vi "loadEthernetRange.vi"(6 "type":string, 8 "error in (no error)":errorcluster, 9 "device.lvclass":refnum<class "device.lvclass">, 10 "xml in":refnum<class "NativeXML.lvclass">, 11 "deviceDataBase in":refnum<class "deviceDataBase.lvclass">) -> (0 "error out":errorcluster, 1 "device.lvclass out":refnum<class "device.lvclass">, 2 "xml out":refnum<class "NativeXML.lvclass">, 3 "deviceDataBase out":refnum<class "deviceDataBase.lvclass">)   [LabVIEW 2011, in "Tools.lvlib" / "DatabaseHelpers.lvlib" / "deviceDataBase.lvclass"]
uses:
  deviceDataBase.lvclass
  NativeXML/NativeXML.lvclass
  Database Objects/device/device.lvclass
  Database Objects/device/EthernetSupply/ethernetSupply.lvclass
  Database Objects/device/AnalogDevice/AnalogDevice.lvclass
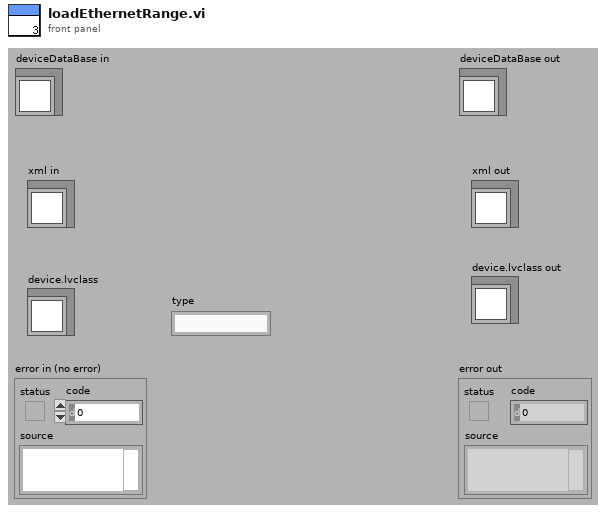
[diagram p1: front panel]
types:
  T1 = cluster{"Range":cluster{"units":string, "current":dbl, "voltage":dbl}, "triggering_inUse":cluster{"start_trigger":string, "clock":string}, "Limits":cluster{"VoltageLimit":dbl, "CurrentLimit":dbl}}[]
  T2 = cluster{"Range":cluster{"units":string, "current":dbl, "voltage":dbl}, "triggering_inUse":cluster{"start_trigger":string, "clock":string}, "Limits":cluster{"VoltageLimit":dbl, "CurrentLimit":dbl}}
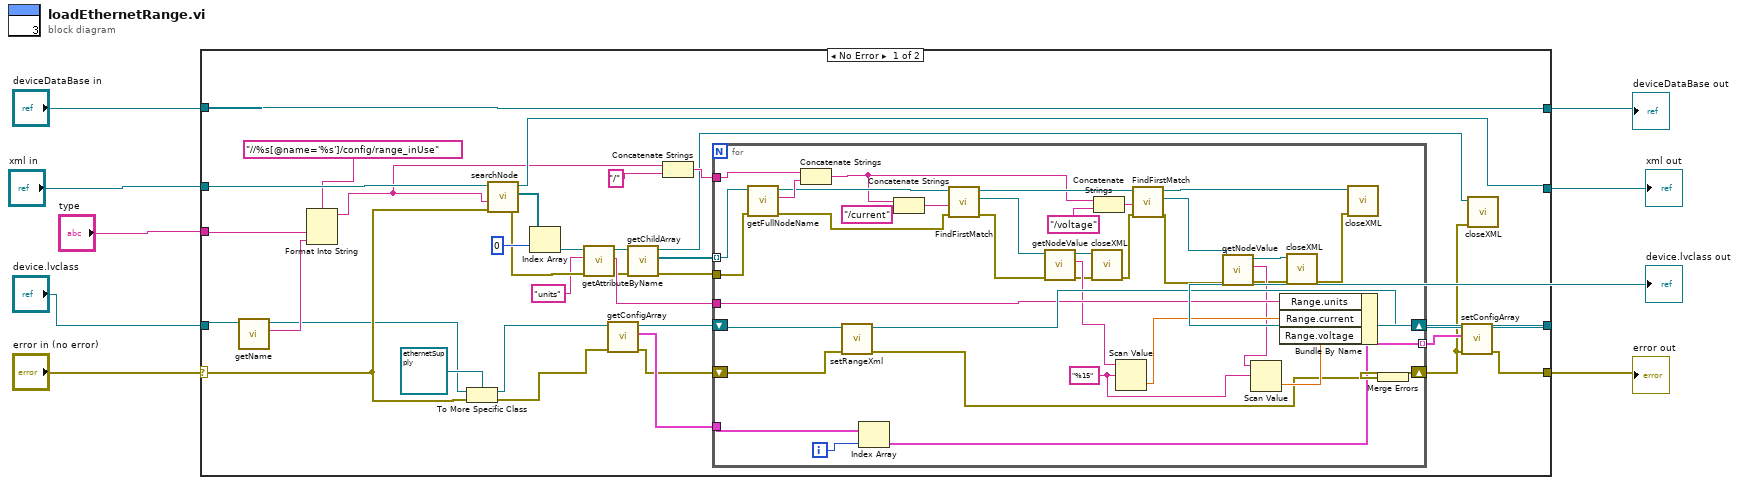
[diagram p0: block diagram]
diagram:
  n1 = case shown="No Error" "error in (no error)" {
    selector: "error in (no error)" -> [w19 w85]
    tunnel: [w33 w85] -> w2
    tunnel: [w43 w84] -> w5
    tunnel: "xml in" -> [w29 w83]
    tunnel: "device.lvclass" -> [w20 w82]
    tunnel: [w34 w82] -> w3
    tunnel: [w30 w83] -> w4
    tunnel: "deviceDataBase in" -> [w43 w84]
    tunnel: "type" -> [w18 _]
    frame No Error {
      n2 = call "getName.vi"("device.lvclass in"=w20) -> ("name"=w17:string, "device.lvclass out"=w16:refnum<class "device.lvclass">)  [unwired: 8 in, 1 out]
      n3 = Format Into String(format string="//%s[@name='%s']/config/range_inUse", w18, w17) -> (resulting string=w10:string)  [unwired: 2 in, 1 out]
      n4 = To More Specific Class(target class=refnum<class "ethernetSupply.lvclass"> refnum ("Tools.lvlib:DatabaseHelpers.lvlib:EthernetSupply.lvclass"), reference=w16, error in=w19) -> (specific class reference=w38:refnum<class "ethernetSupply.lvclass">, error out=w32:errorcluster)
      n5 = call "searchNode.vi"("error in (no error)"=w19, "searchXPath"=w10, "NativeXML in"=w29) -> ("error out"=w28:errorcluster, "nodeArray"=w31:refnum<class "NativeXML.lvclass">[], "NativeXML out"=w30:refnum<class "NativeXML.lvclass">)  [unwired: 6 in]
      n6 = Index Array(array=w31, index=0) -> (element=w26:refnum<class "NativeXML.lvclass">)
      n7 = call "getAttributeByName.vi"("error in (no error)"=w28, "name"="units", "NativeXML in"=w26) -> ("error out"=w23:errorcluster, "Attribute String"=w25:string, "NativeXML out"=w22:refnum<class "NativeXML.lvclass">)  [unwired: 6 in]
      n8 = call "getConfigArray.vi"("error in (no error)"=w32, "EthernetSupply in"=w38) -> ("error out"=w36:errorcluster, "ConfigArray"=w37:T1, "EthernetSupply out"=w39:refnum<class "ethernetSupply.lvclass">)  [unwired: 7 in]
      n9 = call "getChildArray.vi"("error in (no error)"=w23, "NativeXML in"=w22) -> ("error out"=w24:errorcluster, "childArray"=w21:refnum<class "NativeXML.lvclass">[], "NativeXML out"=w13:refnum<class "NativeXML.lvclass">)  [unwired: 7 in]
      n10 = Concatenate Strings(w10, "/") -> (w14:string)
      n11 = for {
        shift-right: [w76] -> w35
        shift-left: w39 -> [w78]
        shift-right: [w74] -> w12
        shift-left: w36 -> [w77]
        tunnel: w21 -> [w66] mode=indexing
        tunnel: [w75] -> w40 mode=indexing
        tunnel: w37 -> [w72]
        tunnel: w24 -> [w60]
        tunnel: w25 -> [w69]
        tunnel: w14 -> [w65]
        i -> [w73]
        w80 = "%15"
        n12 = call "getFullNodeName.vi"("error in (no error)"=w60, "NativeXML in"=w66) -> ("error out"=w56:errorcluster, "fullName"=w64:string, "NativeXML out"=w57:refnum<class "NativeXML.lvclass">)  [unwired: 7 in]
        n13 = Concatenate Strings(w65, w64) -> (w44:string)
        n14 = call "setRangeXml.vi"("error in (no error)"=w77, "AnalogDevice in"=w78) -> ("error out"=w70:errorcluster, "AnalogDevice out"=w76:refnum<class "ethernetSupply.lvclass">)  [unwired: 8 in]
        n15 = Index Array(array=w72, index=w73) -> (element=w71:T2)
        n16 = Concatenate Strings(w44, "/current") -> (w53:string)
        n17 = call "FindFirstMatch.vi"("error in (no error)"=w56, "xPath"=w53, "NativeXML in"=w57) -> ("error out"=w55:errorcluster, "NativeXML match"=w54:refnum<class "NativeXML.lvclass">, "NativeXML out"=w50:refnum<class "NativeXML.lvclass">)  [unwired: 6 in]
        n18 = call "getNodeValue.vi"("error in (no error)"=w55, "NativeXML in"=w54) -> ("error out"=w59:errorcluster, "Value"=w68:string, "NativeXML out"=w58:refnum<class "NativeXML.lvclass">)  [unwired: 7 in]
        n19 = call "closeXML.vi"("error in (no error)"=w59, "NativeXML in"=w58) -> ("error out"=w49:errorcluster)  [unwired: 9 in]
        n20 = Concatenate Strings(w44, "/voltage") -> (w46:string)
        n21 = Scan Value(string=w68, format string=w80) -> (value=w81:dbl)  [unwired: 1 in, 1 out]
        n22 = call "FindFirstMatch.vi"("error in (no error)"=w49, "xPath"=w46, "NativeXML in"=w50) -> ("error out"=w48:errorcluster, "NativeXML match"=w47:refnum<class "NativeXML.lvclass">, "NativeXML out"=w51:refnum<class "NativeXML.lvclass">)  [unwired: 6 in]
        n23 = call "getNodeValue.vi"("error in (no error)"=w48, "NativeXML in"=w47) -> ("error out"=w63:errorcluster, "Value"=w67:string, "NativeXML out"=w62:refnum<class "NativeXML.lvclass">)  [unwired: 7 in]
        n24 = Scan Value(string=w67, format string=w80) -> (value=w79:dbl)  [unwired: 1 in, 1 out]
        n25 = Bundle By Name(cluster=w71, "Range.units"=w69, "Range.current"=w81, "Range.voltage"=w79) -> (w75:T2)
        n26 = call "closeXML.vi"("error in (no error)"=w63, "NativeXML in"=w62) -> ("error out"=w61:errorcluster)  [unwired: 9 in]
        n27 = call "closeXML.vi"("error in (no error)"=w61, "NativeXML in"=w51) -> ()  [unwired: 9 in, 1 out]
        n28 = Merge Errors(w70) -> (w74:errorcluster)
      }
      n29 = call "setConfigArray.vi"("error in (no error)"=w12, "ConfigArray"=w40, "EthernetSupply in"=w35) -> ("error out"=w33:errorcluster, "EthernetSupply out"=w34:refnum<class "ethernetSupply.lvclass">)  [unwired: 7 in]
      n30 = call "closeXML.vi"("error in (no error)"=w12, "NativeXML in"=w13) -> ()  [unwired: 9 in, 1 out]
    }
    frame Error {
    }
  }
  "error out" <- w2
  "deviceDataBase out" <- w5
  "xml out" <- w4
  "device.lvclass out" <- w3
